vi "Format Number for Table.vi"(6 "HTML Color":string, 9 "Number":dbl) -> (1 "Number String":string)   [LabVIEW 2011]
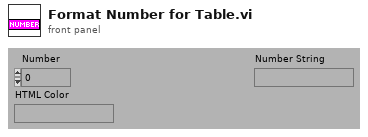
[diagram p1: front panel]
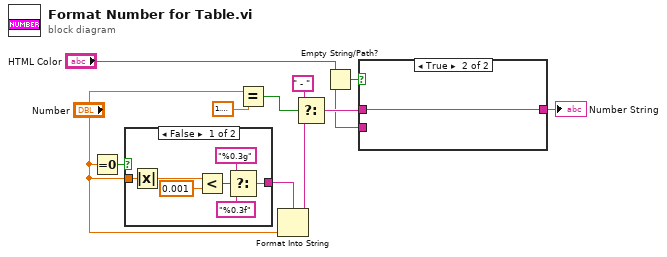
[diagram p0: block diagram]
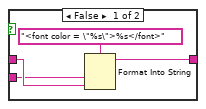
[diagram p2: hidden frame]
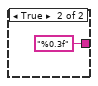
[diagram p3: hidden frame]
diagram:
  n1 = Equal To 0?(x="Number") -> (x = 0?=w8:bool)
  n2 = case shown="False" w8 {
    tunnel: "Number" -> [w18 _]
    tunnel: [w14 "%0.3f" ("search string")] -> w9
    frame False {
      n3 = Absolute Value(x=w18) -> (abs(x)=w12:dbl)
      n4 = Less?(x=w12, y=0.001) -> (x < y?=w16:bool)
      n5 = Select(t="%0.3g" ("search string"), s=w16, f="%0.3f" ("search string")) -> (s? t:f=w14:string)
    }
    frame True {
    }
  }
  n6 = Equal?(x="Number", y=1.1447298858494002) -> (x = y?=w1:bool)
  n7 = Format Into String(format string=w9, "Number") -> (resulting string=w10:string)  [unwired: 2 in, 1 out]
  n8 = Select(t=" - " ("search string"), s=w1, f=w10) -> (s? t:f=w6:string)
  n9 = Empty String/Path?(string/path="HTML Color") -> (empty?=w7:bool)
  n10 = case shown="True" w7 {
    tunnel: w6 -> [w21 w24]
    tunnel: [w22 w24] -> w5
    tunnel: "HTML Color" -> [w20 _]
    frame False {
      n11 = Format Into String(format string="<font color = \"%s\">%s</font>" ("search string"), w20, w21) -> (resulting string=w22:string)  [unwired: 2 in, 1 out]
    }
    frame True {
    }
  }
  "Number String" <- w5
